vi "table名称.vi"(11 "设备名称":string="Screw_Machine") -> (2 "ERtable":string, 3 "IOTtable":string)   [LabVIEW 2017]
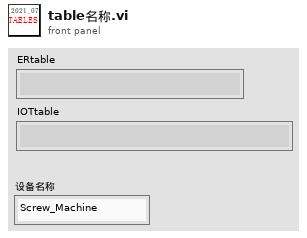
[diagram p1: front panel]
types:
  T1 = cluster{"%Y_%m_%d_%H_%M_%S%3u":string, "%Y_%m_%d":string, "%H_%M_%S%3u":string}
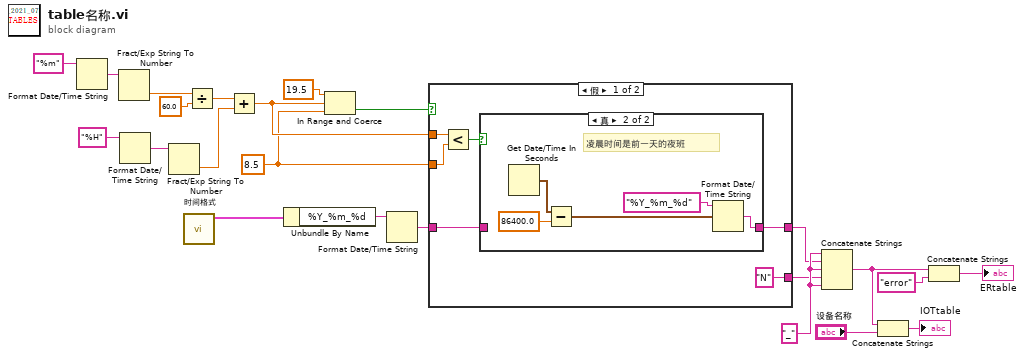
[diagram p0: block diagram]
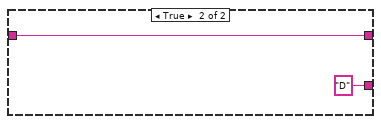
[diagram p3: hidden frame]
diagram:
  w22 = "_" ("时间格式字符串(%c)")
  w1 = 8.5 ("下限")
  n1 = Format Date/Time String(time format string (%c)="%m" ("时间格式字符串(%c)")) -> (date/time string=w7:string)  [unwired: 2 in]
  n2 = Fract/Exp String To Number(string=w7) -> (number=w9:dbl)  [unwired: 3 in, 1 out]
  n3 = Format Date/Time String(time format string (%c)="%H" ("时间格式字符串(%c)")) -> (date/time string=w5:string)  [unwired: 2 in]
  n4 = Fract/Exp String To Number(string=w5) -> (number=w3:dbl)  [unwired: 3 in, 1 out]
  n5 = call "时间格式.vi"() -> ("时间格式"=w13:T1)  [unwired: 11 in]
  n6 = Divide(x=w9, y=60.0) -> (x/y=w4:dbl)
  n7 = Add(x=w4, y=w3) -> (x+y=w2:dbl)
  n8 = Unbundle By Name ("按名称解除捆绑")(w13) -> ("%Y_%m_%d"=w14:string)
  n9 = In Range and Coerce(upper limit=19.5 ("上限"), x=w2, lower limit=w1) -> (In Range?=w16:bool)  [unwired: 1 out]
  n10 = Format Date/Time String(time format string (%c)=w14) -> (date/time string=w11:string)  [unwired: 2 in]
  n11 = case shown="假" w16 {
    tunnel: ["N" ("时间格式字符串(%c)") "D" ("时间格式字符串(%c)")] -> w15
    tunnel: w2 -> [w29 _]
    tunnel: [w26 w36] -> w12
    tunnel: w11 -> [w25 w36]
    tunnel: w1 -> [w24 _]
    frame False {
      n12 = Less?(x=w29, y=w24) -> (x < y?=w28:bool)
      n13 = case shown="真" w28 {
        tunnel: [w30 w31] -> w26
        tunnel: w25 -> [w30 _]
        frame False {
        }
        frame True {
          # "凌晨时间是前一天的夜班"
          n14 = Get Date/Time In Seconds() -> (seconds since 1Jan1904=w34:timestamp)
          n15 = Subtract(x=w34, y=86400.0) -> (x-y=w35:timestamp)
          n16 = Format Date/Time String(time format string (%c)="%Y_%m_%d" ("时间格式字符串(%c)"), seconds (now)=w35) -> (date/time string=w31:string)  [unwired: 1 in]
        }
      }
    }
    frame True {
    }
  }
  n17 = Concatenate Strings(w22, w12, w22, w15, w22) -> (w19:string)
  n18 = Concatenate Strings(w19, "设备名称") -> (→"IOTtable":string)
  n19 = Concatenate Strings(w19, "error" ("字符串")) -> (→"ERtable":string)
